vi "RT Error Handler - UI Commands.vi"(8 "error in (no error)":errorcluster caption="错误输入（无错误）", 11 "Message Queue":refnum<queue> caption="消息队列") -> (3 "dup Message Queue":refnum<queue> caption="消息队列副本")   [LabVIEW 2013]
uses:
  support/Message Queue/Message Cluster.ctl
  support/Message Queue/Message Queue.lvlib
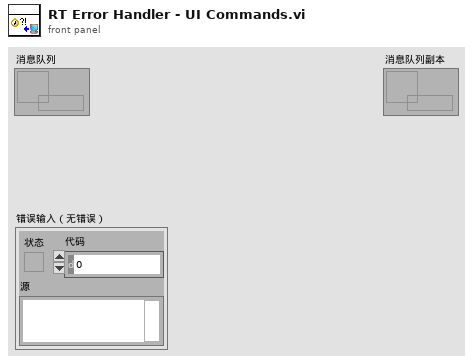
[diagram p1: front panel]
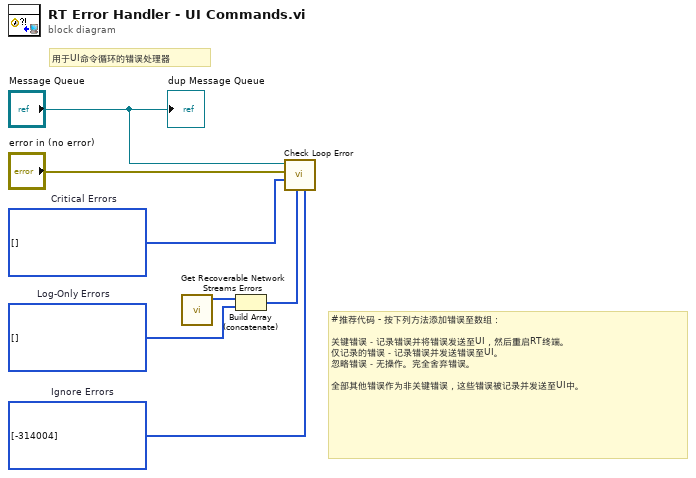
[diagram p0: block diagram]
diagram:
  w6 = i32[] [-314004]  # Ignore Errors
  w2 = i32[] []  # Log-Only Errors
  w7 = i32[] []  # Critical Errors
  # "#推荐代码 - 按下列方法添加错误至数组：\n\n关键错误－记录错误并将错误发送至UI，然后重启RT终端。\n仅记录的错误－记录错误并发送错误至UI。\n忽略错误－无操作。完全舍弃错误。\n\n全部其他错误作为非关键错误，这些错误被记录并发送至UI中。"
  # "用于UI命令循环的错误处理器"
  n1 = call "Get Recoverable Network Streams Errors.vi"() -> ("recoverable network streams errors"=w3:i32[])  [unwired: 11 in]
  n2 = Build Array (concatenate)(w3, w2) -> (w1:i32[])
  n3 = call "Check Loop Error.vi"("Ignore Errors"=w6, "Log-Only Errors"=w1, "Critical Errors"=w7, "error to process"="error in (no error)", "Message Queue"="Message Queue") -> ()  [unwired: 5 in, 2 out]
  "dup Message Queue" <- "Message Queue"
